vi "Move.vi"(8 "error in (no error)":errorcluster, 9 "Absolute (T)":bool=TRUE, 10 "Point":refnum<class "Point.lvclass">, 11 "Shape in":refnum<class "Shape.lvclass">) -> (0 "error out":errorcluster, 3 "Shape out":refnum<class "Shape.lvclass">)   [LabVIEW 2021, in "Picture2D.lvlib" / "Shape.lvclass"]
uses:
  Shape.lvclass
  Point/Point.lvclass
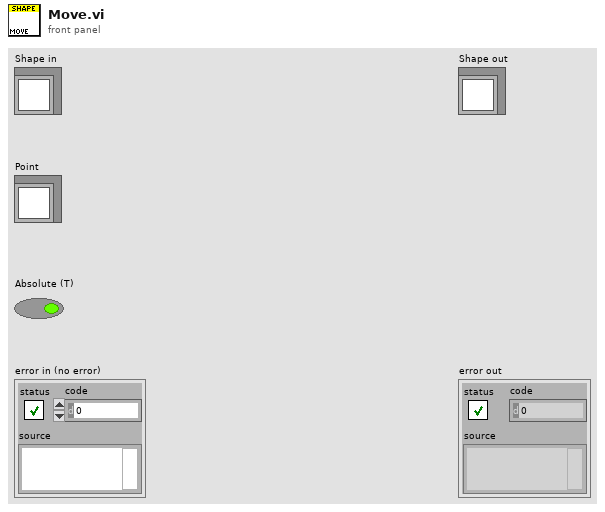
[diagram p1: front panel]
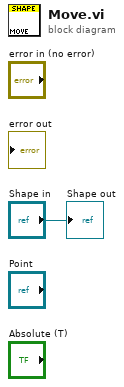
[diagram p0: block diagram]
diagram:
  "Shape out" <- "Shape in"
